vi "Mason Messy Teleop.vi"   [LabVIEW 2017]
doc: "This VI is called for each TeleOp packet received from the DS where the robot is not disabled. It is often used to read from the joysticks and update I/O or to update setpoints for timed control loops. It should complete and return within 20 milliseconds or it may miss DS packets."
uses:
  Systems/MechamumDrive/Cluster_CMD to SM Data.ctl
  Systems/MechamumDrive/Enum_SM Cmd Select.ctl
  Joystick/Enum_SingleStickAxes.ctl
  Systems/Intake/Cluster_Cmd to SM Data.ctl
  Systems/Intake/Enum_SM Cmd Select.ctl
  Systems/Shooter/Cluster_CMD to SM Data.ctl
  Systems/Shooter/ENUM_CMD Select.ctl
  Systems/Climber/Cluster_Cmd to SM Data.ctl
  Systems/Climber/ENUM_SM Cmd Select.ctl
  Systems/VisionSystem/Cluster_CMD to Vision.ctl
  Systems/VisionSystem/Enum_ Field Targets.ctl
  <vilib>/Rock Robotics/WPI/Solenoid/WPI_SolenoidValue.ctl
  Systems/Controller/Global_Data Out.vi
  Systems/Controller/Global Control Outputs.vi
  Systems/Hopper/Global_SM_Data Out.vi
  Systems/Climber/Global_CMD to SM Data.vi
  Systems/VisionSystem/Global_CMD Data.vi
  Systems/Gear/Global_GearPistonsCTRL.vi
  Systems/Intake/Global_CMD to SM Data.vi
  Systems/Shooter/Global_CMD to SM Data.vi
  Systems/MechamumDrive/Global_CMD to SM Data.vi
  Systems/MechamumDrive/MechamunDrive.lvlib
  Joystick/Joystick.lvlib
  Systems/Intake/Intake.lvlib
  Systems/Controller/Controller.lvlib
  Systems/Hopper/Hopper System.lvlib
  Systems/Shooter/Shooter.lvlib
  Systems/Climber/Climber.lvlib
  Systems/Gear/Gear.lvlib
  Systems/VisionSystem/VisionSystem.lvlib
types:
  T1 = typedef "VisionSystem.lvlib/Cluster_CMD to Vision.ctl" = cluster{"CMD_Target":T2}
  T2 = typedef "VisionSystem.lvlib/Enum_ Field Targets.ctl" = enum16{"Boiler (USB 0)", "Rope (USB 1)"}
  T3 = typedef "Climber.lvlib/Cluster_Cmd to SM Data.ctl" = cluster{"Climber Command Mode":T4}
  T4 = typedef "Climber.lvlib/ENUM_SM Cmd Select.ctl" = enum16{"Stop", "Auto Climb", "Manual", "No Command"}
  T5 = typedef "Shooter.lvlib/Cluster_CMD to SM Data.ctl" = cluster{"Select":T6, "Wheel VBus":dbl, "Wheel RPM":dbl, "Hood VBus":dbl, "Hood Position":dbl}
  T6 = typedef "Shooter.lvlib/ENUM_CMD Select.ctl" = enum16{"Stop", "Manual VBus", "Encoder Hood Only", "Encoder Wheel Only", "Encoder Both"}
  T7 = typedef "Intake.lvlib/Cluster_Cmd to SM Data.ctl" = cluster{"Intake Mode":T8, "VBus":dbl}
  T8 = typedef "Intake.lvlib/Enum_SM Cmd Select.ctl" = enum16{"No Command", "Manual", "Half Speed", "Full Speed", "Reverse", "Stop"}
  T9 = typedef "Joystick.lvlib/Enum_SingleStickAxes.ctl" = enum16{"X-Axis (-1 to 1)", "Y-Axis (-1 to 1)", "Z-Axis Rotation (-1 to 1)", "Slider (0 to 1)"}
  T10 = typedef "MechamunDrive.lvlib/Cluster_CMD to SM Data.ctl" = cluster{"CMDMODE":T11, "X":dbl, "Y":dbl, "Rotation":dbl, "Auto Angle":dbl, "Speed Divider":dbl, "Use Gyro":bool, "Target Distance":dbl}
  T11 = typedef "MechamunDrive.lvlib/Enum_SM Cmd Select.ctl" = enum16{"No Command", "Halt", "Manual Keep Rotation", "Manual", "Track Front", "Track Rotation", "Track Lateral", "Track Vision Lat", "Track Vision Rot", "Strafe Right", "Strafe Left"}
  T12 = typedef "WPI_SolenoidValue.ctl" = enum16{"Off", "On", "Forward", "Reverse"}
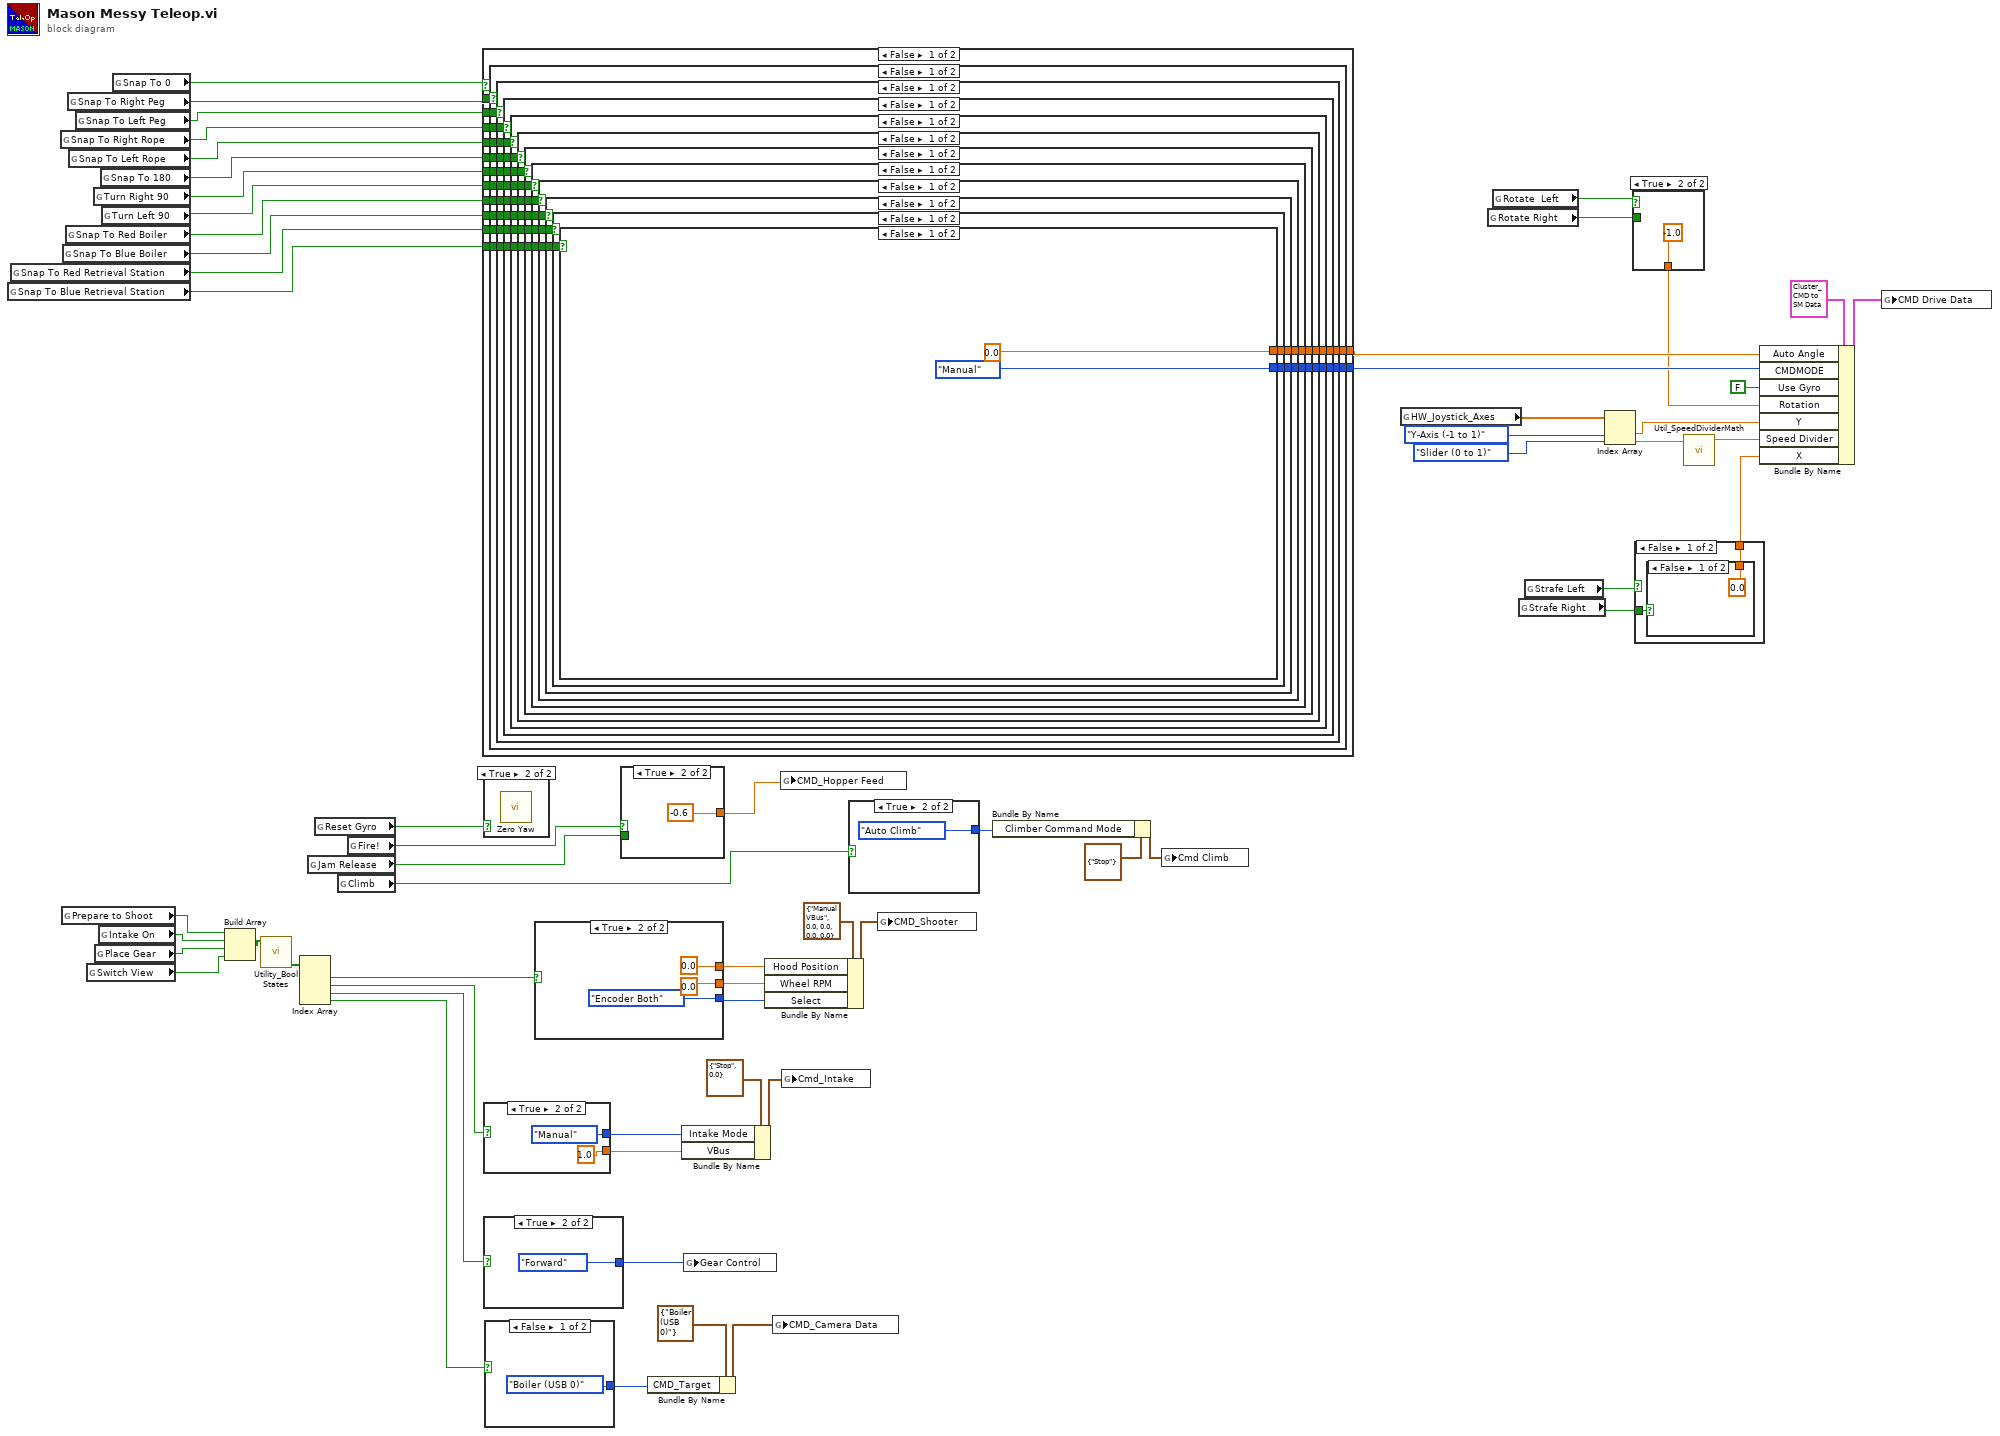
[diagram p0: block diagram]
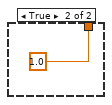
[diagram p2: hidden frame]
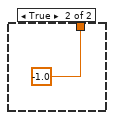
[diagram p3: hidden frame]
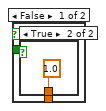
[diagram p4: hidden frame]
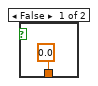
[diagram p5: hidden frame]
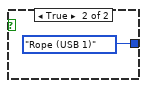
[diagram p6: hidden frame]
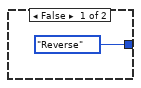
[diagram p7: hidden frame]
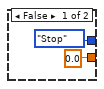
[diagram p8: hidden frame]
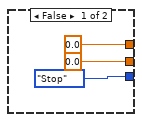
[diagram p9: hidden frame]
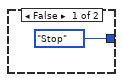
[diagram p10: hidden frame]
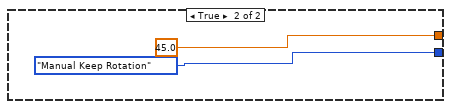
[diagram p11: hidden frame]
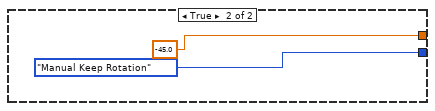
[diagram p12: hidden frame]
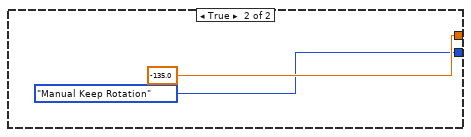
[diagram p13: hidden frame]
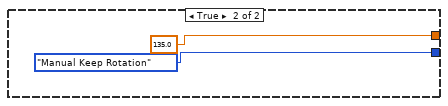
[diagram p14: hidden frame]
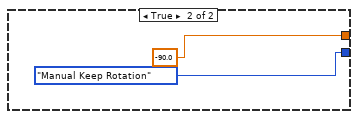
[diagram p15: hidden frame]
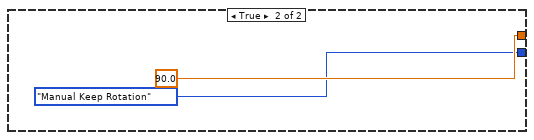
[diagram p16: hidden frame]
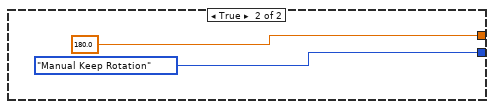
[diagram p17: hidden frame]
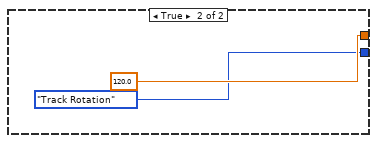
[diagram p18: hidden frame]
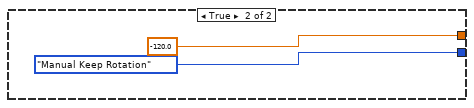
[diagram p19: hidden frame]
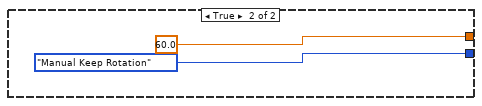
[diagram p20: hidden frame]
diagram:
  n1 = global read "Global Control Outputs.vi" "Snap To Blue Retrieval Station"() -> (w27:bool)
  n2 = global read "Global Control Outputs.vi" "Snap To Red Retrieval Station"() -> (w28:bool)
  n3 = global read "Global Control Outputs.vi" "Snap To Right Rope"() -> (w35:bool)
  n4 = global read "Global Control Outputs.vi" "Prepare to Shoot"() -> (w21:bool)
  n5 = global read "Global Control Outputs.vi" "Snap To Blue Boiler"() -> (w29:bool)
  n6 = global read "Global Control Outputs.vi" "Snap To Red Boiler"() -> (w30:bool)
  n7 = global read "Global Control Outputs.vi" "Snap To Right Peg"() -> (w37:bool)
  n8 = global read "Global Control Outputs.vi" "Snap To Left Rope"() -> (w34:bool)
  n9 = global read "Global Control Outputs.vi" "Snap To Left Peg"() -> (w36:bool)
  n10 = global read "Global Control Outputs.vi" "Switch View"() -> (w17:bool)
  n11 = global read "Global Control Outputs.vi" "Turn Right 90"() -> (w32:bool)
  n12 = global read "Global Control Outputs.vi" "Place Gear"() -> (w23:bool)
  n13 = global read "Global Control Outputs.vi" "Intake On"() -> (w22:bool)
  n14 = global read "Global Control Outputs.vi" "Snap To 180"() -> (w33:bool)
  n15 = global read "Global Control Outputs.vi" "Turn Left 90"() -> (w31:bool)
  n16 = global read "Global Control Outputs.vi" "Snap To 0"() -> (w38:bool)
  n17 = Build Array(w21, w22, w23, w17) -> (w20:bool[])
  n18 = call "Utility_Bool States.vi"("HW_Joystick_Buttons"=w20) -> ("Toggle On Rizing Out"=w47:bool[])  [unwired: 6 in, 4 out]
  n19 = Index Array(array=w47) -> (element #1=w19:bool, element #2=w51:bool, element #3=w48:bool, element #4=w16:bool)  [unwired: 4 in]
  n20 = global read "Global Control Outputs.vi" "Jam Release"() -> (w25:bool)
  n21 = global read "Global Control Outputs.vi" "Reset Gyro"() -> (w26:bool)
  n22 = global read "Global Control Outputs.vi" "Climb"() -> (w24:bool)
  n23 = global read "Global Control Outputs.vi" "Fire!"() -> (w18:bool)
  n24 = case shown="False" w38 {
    tunnel: w37 -> [w73 _]
    tunnel: w36 -> [w72 _]
    tunnel: w35 -> [w71 _]
    tunnel: w34 -> [w70 _]
    tunnel: w33 -> [w69 _]
    tunnel: w32 -> [w68 _]
    tunnel: w31 -> [w67 _]
    tunnel: w30 -> [w66 _]
    tunnel: w29 -> [w65 _]
    tunnel: w28 -> [w64 _]
    tunnel: w27 -> [w63 _]
    tunnel: [w62 0.0 ("Auto Angle")] -> w54
    tunnel: [w61 Enum_SM_Cmd_Select."Manual Keep Rotation" ("CMDMODE")] -> w55
    frame False {
      n25 = case shown="False" w73 {
        tunnel: w72 -> [w85 _]
        tunnel: w71 -> [w84 _]
        tunnel: w70 -> [w83 _]
        tunnel: w69 -> [w82 _]
        tunnel: w68 -> [w81 _]
        tunnel: w67 -> [w80 _]
        tunnel: w66 -> [w79 _]
        tunnel: w65 -> [w78 _]
        tunnel: w64 -> [w77 _]
        tunnel: w63 -> [w76 _]
        tunnel: [w75 -60.0 ("Auto Angle")] -> w62
        tunnel: [w74 Enum_SM_Cmd_Select."Manual Keep Rotation" ("CMDMODE")] -> w61
        frame False {
          n26 = case shown="False" w85 {
            tunnel: w84 -> [w96 _]
            tunnel: w83 -> [w95 _]
            tunnel: w82 -> [w94 _]
            tunnel: w81 -> [w93 _]
            tunnel: w80 -> [w92 _]
            tunnel: w79 -> [w91 _]
            tunnel: w78 -> [w90 _]
            tunnel: w77 -> [w89 _]
            tunnel: w76 -> [w88 _]
            tunnel: [w87 60.0 ("Auto Angle")] -> w75
            tunnel: [w86 Enum_SM_Cmd_Select."Manual Keep Rotation" ("CMDMODE")] -> w74
            frame False {
              n27 = case shown="False" w96 {
                tunnel: w95 -> [w106 _]
                tunnel: w94 -> [w105 _]
                tunnel: w93 -> [w104 _]
                tunnel: w92 -> [w103 _]
                tunnel: w91 -> [w102 _]
                tunnel: w90 -> [w101 _]
                tunnel: w89 -> [w100 _]
                tunnel: w88 -> [w99 _]
                tunnel: [w98 -120.0 ("Auto Angle")] -> w87
                tunnel: [w97 Enum_SM_Cmd_Select."Manual Keep Rotation" ("CMDMODE")] -> w86
                frame False {
                  n28 = case shown="False" w106 {
                    tunnel: w105 -> [w115 _]
                    tunnel: w104 -> [w114 _]
                    tunnel: w103 -> [w113 _]
                    tunnel: w102 -> [w112 _]
                    tunnel: w101 -> [w111 _]
                    tunnel: w100 -> [w110 _]
                    tunnel: w99 -> [w109 _]
                    tunnel: [w108 120.0 ("Auto Angle")] -> w98
                    tunnel: [w107 Enum_SM_Cmd_Select."Track Rotation" ("CMDMODE")] -> w97
                    frame False {
                      n29 = case shown="False" w115 {
                        tunnel: w114 -> [w123 _]
                        tunnel: w113 -> [w122 _]
                        tunnel: w112 -> [w121 _]
                        tunnel: w111 -> [w120 _]
                        tunnel: w110 -> [w119 _]
                        tunnel: w109 -> [w118 _]
                        tunnel: [w117 180.0 ("Auto Angle")] -> w108
                        tunnel: [w116 Enum_SM_Cmd_Select."Manual Keep Rotation" ("CMDMODE")] -> w107
                        frame False {
                          n30 = case shown="False" w123 {
                            tunnel: w122 -> [w130 _]
                            tunnel: w121 -> [w129 _]
                            tunnel: w120 -> [w128 _]
                            tunnel: w119 -> [w127 _]
                            tunnel: w118 -> [w126 _]
                            tunnel: [w125 90.0 ("Auto Angle")] -> w117
                            tunnel: [w124 Enum_SM_Cmd_Select."Manual Keep Rotation" ("CMDMODE")] -> w116
                            frame False {
                              n31 = case shown="False" w130 {
                                tunnel: w129 -> [w136 _]
                                tunnel: w128 -> [w135 _]
                                tunnel: w127 -> [w134 _]
                                tunnel: w126 -> [w133 _]
                                tunnel: [w132 -90.0 ("Auto Angle")] -> w125
                                tunnel: [w131 Enum_SM_Cmd_Select."Manual Keep Rotation" ("CMDMODE")] -> w124
                                frame False {
                                n32 = case shown="False" w136 {
                                tunnel: w135 -> [w141 _]
                                tunnel: w134 -> [w140 _]
                                tunnel: w133 -> [w139 _]
                                tunnel: [w138 135.0 ("Auto Angle")] -> w132
                                tunnel: [w137 Enum_SM_Cmd_Select."Manual Keep Rotation" ("CMDMODE")] -> w131
                                frame False {
                                n33 = case shown="False" w141 {
                                tunnel: w140 -> [w145 _]
                                tunnel: w139 -> [w144 _]
                                tunnel: [w143 -135.0 ("Auto Angle")] -> w138
                                tunnel: [w142 Enum_SM_Cmd_Select."Manual Keep Rotation" ("CMDMODE")] -> w137
                                frame False {
                                n34 = case shown="False" w145 {
                                tunnel: w144 -> [w148 _]
                                tunnel: [w147 -45.0 ("Auto Angle")] -> w143
                                tunnel: [w146 Enum_SM_Cmd_Select."Manual Keep Rotation" ("CMDMODE")] -> w142
                                frame False {
                                n35 = case shown="False" w148 {
                                tunnel: [0.0 ("Auto Angle") 45.0 ("Auto Angle")] -> w147
                                tunnel: [Enum_SM_Cmd_Select."Manual" ("CMDMODE") Enum_SM_Cmd_Select."Manual Keep Rotation" ("CMDMODE")] -> w146
                                frame False {
                                }
                                frame True {
                                }
                                }
                                }
                                frame True {
                                }
                                }
                                }
                                frame True {
                                }
                                }
                                }
                                frame True {
                                }
                                }
                                }
                                frame True {
                                }
                              }
                            }
                            frame True {
                            }
                          }
                        }
                        frame True {
                        }
                      }
                    }
                    frame True {
                    }
                  }
                }
                frame True {
                }
              }
            }
            frame True {
            }
          }
        }
        frame True {
        }
      }
    }
    frame True {
    }
  }
  n36 = case shown="True" w26 {
    frame False {
    }
    frame True {
      n37 = call <vilib>:"Zero Yaw.vi"() -> ()  [unwired: 12 in]
    }
  }
  n38 = case shown="True" w51 {
    tunnel: [0.0 ("VBus") 1.0 ("VBus")] -> w50
    tunnel: [Enum_SM_Cmd_Select."Stop" ("Intake Mode") Enum_SM_Cmd_Select."Manual" ("Intake Mode")] -> w49
    frame False {
    }
    frame True {
    }
  }
  n39 = case shown="True" w48 {
    tunnel: [WPI_SolenoidValue."Reverse" ("Gear Control") WPI_SolenoidValue."Forward" ("Gear Control")] -> w39
    frame False {
    }
    frame True {
    }
  }
  n40 = case shown="False" w16 {
    tunnel: [Enum__Field_Targets."Boiler (USB 0)" ("CMD_Target") Enum__Field_Targets."Rope (USB 1)" ("CMD_Target")] -> w13
    frame False {
    }
    frame True {
    }
  }
  n41 = case shown="True" w19 {
    tunnel: [ENUM_CMD_Select."Stop" ("Select") ENUM_CMD_Select."Encoder Both" ("Select")] -> w45
    tunnel: [0.0 ("Hood Position") 0.0 ("Hood Position")] -> w44
    tunnel: [0.0 ("Wheel RPM") 0.0 ("Hood Position")] -> w43
    frame False {
    }
    frame True {
    }
  }
  n42 = case shown="True" w18 {
    tunnel: [w189 -0.6 ("Hopper")] -> w10
    tunnel: w25 -> [w190 _]
    frame False {
      n43 = case shown="False" w190 {
        tunnel: [0.0 ("Hopper") 0.7 ("Hopper")] -> w189
        frame False {
        }
        frame True {
        }
      }
    }
    frame True {
    }
  }
  n44 = Bundle By Name(cluster=T1 {"CMD_Target"=enum."Boiler (USB 0)"} ("CMD_Camera Data"), "CMD_Target"=w13) -> (w14:T1)
  n45 = Bundle By Name(cluster=T7 {"Intake Mode"=enum."Stop", "VBus"=0.0} ("Intake"), "Intake Mode"=w49, "VBus"=w50) -> (w52:T7)
  n46 = global write "Global_GearPistonsCTRL.vi" "Gear Control"(w39) -> ()
  n47 = Bundle By Name(cluster=T5 {"Select"=enum."Manual VBus", "Wheel VBus"=0.0, "Wheel RPM"=0.0, "Hood VBus"=0.0, "Hood Position"=0.0} ("CMD_Shooter"), "Hood Position"=w44, "Wheel RPM"=w43, "Select"=w45) -> (w9:T5)
  n48 = global write "Global_CMD Data.vi" "CMD_Camera Data"(w14) -> ()
  n49 = global write "Global_SM_Data Out.vi" "CMD_Hopper Feed"(w10) -> ()
  n50 = global write "Global_CMD to SM Data.vi" "Cmd_Intake"(w52) -> ()
  n51 = case shown="True" w24 {
    tunnel: [ENUM_SM_Cmd_Select."Stop" ("Climber Command Mode") ENUM_SM_Cmd_Select."Auto Climb" ("Climber Command Mode")] -> w40
    frame False {
    }
    frame True {
    }
  }
  n52 = global write "Global_CMD to SM Data.vi" "CMD_Shooter"(w9) -> ()
  n53 = Bundle By Name(cluster=T3 {"Climber Command Mode"=enum."Stop"} ("Cmd Climb"), "Climber Command Mode"=w40) -> (w41:T3)
  n54 = global write "Global_CMD to SM Data.vi" "Cmd Climb"(w41) -> ()
  n55 = global read "Global_Data Out.vi" "HW_Joystick_Axes"() -> (w57:dbl[])
  n56 = global read "Global Control Outputs.vi" "Rotate Right"() -> (w11:bool)
  n57 = global read "Global Control Outputs.vi" "Rotate  Left"() -> (w12:bool)
  n58 = global read "Global Control Outputs.vi" "Strafe Right"() -> (w1:bool)
  n59 = global read "Global Control Outputs.vi" "Strafe Left"() -> (w3:bool)
  n60 = Index Array(array=w57, index #1=Enum_SingleStickAxes."Y-Axis (-1 to 1)", index #2=Enum_SingleStickAxes."Slider (0 to 1)") -> (element #1=w6:dbl, element #2=w5:dbl)
  n61 = case shown="True" w12 {
    tunnel: [w196 -1.0 ("Auto Angle")] -> w4
    tunnel: w11 -> [w197 _]
    frame False {
      n62 = case shown="True" w197 {
        tunnel: [0.0 ("Auto Angle") 1.0 ("Auto Angle")] -> w196
        frame False {
        }
        frame True {
        }
      }
    }
    frame True {
    }
  }
  n63 = case shown="False" w3 {
    tunnel: [w201 -1.0] -> w2
    tunnel: w1 -> [w202 _]
    frame False {
      n64 = case shown="False" w202 {
        tunnel: [0.0 1.0] -> w201
        frame False {
        }
        frame True {
        }
      }
    }
    frame True {
    }
  }
  n65 = call "Util_SpeedDividerMath.vi"("Axis Value"=w5) -> ("Divider Value"=w7:dbl)  [unwired: 10 in]
  n66 = Bundle By Name(cluster=T10 {"CMDMODE"=enum."No Command", "X"=0.0, "Y"=0.0, "Rotation"=0.0, "Auto Angle"=0.0, "Speed Divider"=0.0, "Use Gyro"=FALSE, "Target Distance"=0.0} ("Cmd Drive"), "Auto Angle"=w54, "CMDMODE"=w55, "Use Gyro"=FALSE, "Rotation"=w4, "Y"=w6, "Speed Divider"=w7, "X"=w2) -> (w8:T10)
  n67 = global write "Global_CMD to SM Data.vi" "CMD Drive Data"(w8) -> ()
